vi "Read TriggersTillShot.vi"(8 "error in (no error)":errorcluster, 11 "BME_DG_System in":refnum<class "BME_DG_System.lvclass">) -> (0 "error out":errorcluster, 1 "TriggerCounters":i32[](array[numeric]), 2 "RemainingTriggers":T1(array[cluster]), 3 "BME_DG_System out":refnum<class "BME_DG_System.lvclass">)   [LabVIEW 2009, in "POLARIS BME DG.lvlib" / "BME_DG_System.lvclass"]
uses:
  BME_DG_System.lvclass
  BME_DG_System.lvclass/BME_DG_System.ctl
  BME_DG_Base/BME_DG_Base.lvclass
  BME_DG_Chnl/BME_DG_Chnl.lvclass
panel:
  in  "Cluster":cluster{"Time Stamp":timestamp, "Numeric":i32} {"Time Stamp" format="%<%.3X>T"}
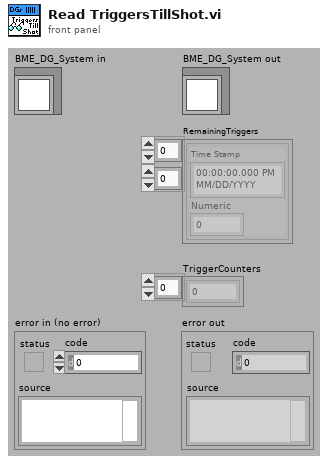
[diagram p1: front panel]
types:
  T1 = cluster{"Time Stamp":timestamp, "Numeric":i32}[][]
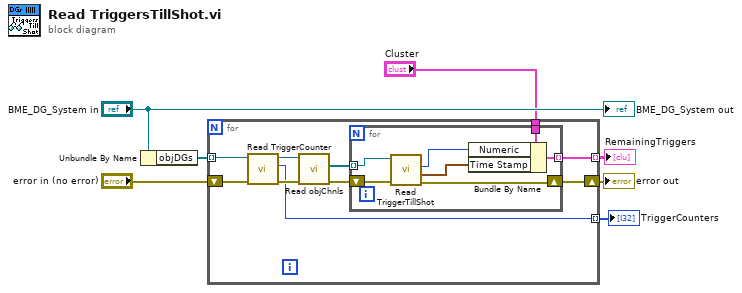
[diagram p0: block diagram]
diagram:
  n1 = Unbundle By Name("BME_DG_System in") -> ("objDGs"=w6:refnum<class "BME_DG_Base.lvclass">[])
  n2 = for {
    tunnel: w6 -> [w12] mode=indexing
    shift-right: [w16] -> w4
    shift-left: "error in (no error)" -> [w10]
    tunnel: "Cluster" -> [w14]
    tunnel: [w13] -> w2 mode=indexing
    tunnel: [w8] -> w1 mode=indexing
    n3 = call "Read TriggerCounter.vi"("error in (no error)"=w10, "BME_DG_Base in"=w12) -> ("error out"=w9:errorcluster, "TriggerCounter"=w8:i32, "BME_DG_Base out"=w11:refnum<class "BME_DG_Base.lvclass">)  [unwired: 7 in]
    n4 = call-dynamic "Read objChnls.vi"("error in (no error)"=w9, "BME_DG_Base in"=w11) -> ("error out"=w17:errorcluster, "objChnls"=w15:refnum<class "BME_DG_Chnl.lvclass">[])  [unwired: 6 in, 2 out]
    n5 = for {
      shift-right: [w22] -> w16
      shift-left: w17 -> [w23]
      tunnel: w15 -> [w24] mode=indexing
      tunnel: w14 -> [w18]
      tunnel: [w19] -> w13 mode=indexing
      n6 = call-dynamic "Read TriggerTillShot.vi"("error in (no error)"=w23, "BME_DG_Chnl in"=w24) -> ("error out"=w22:errorcluster, "LastUpdate"=w21:timestamp, "TriggerTillShot"=w20:i32)  [unwired: 6 in, 1 out]
      n7 = Bundle By Name(cluster=w18, "Numeric"=w20, "Time Stamp"=w21) -> (w19:cluster{"Time Stamp":timestamp, "Numeric":i32})
    }
  }
  "error out" <- w4
  "RemainingTriggers" <- w2
  "TriggerCounters" <- w1
  "BME_DG_System out" <- "BME_DG_System in"
